vi "init.vi"(8 "error in (no error)":errorcluster, 11 "CL57RS in":refnum<class "CL57RS.lvclass">) -> (0 "error out":errorcluster, 3 "CL57RS out":refnum<class "CL57RS.lvclass">)   [LabVIEW 2025, in "Motor.lvlib" / "CL57RS.lvclass"]
uses:
  CL57RS.lvclass
  CL57RS.lvclass/CL57RS.ctl
  <vilib>/NI/Modbus Library/API/Wrapper/Create Serial Master.vi
  <vilib>/NI/Modbus Library/API/Wrapper/API Main.lvlib
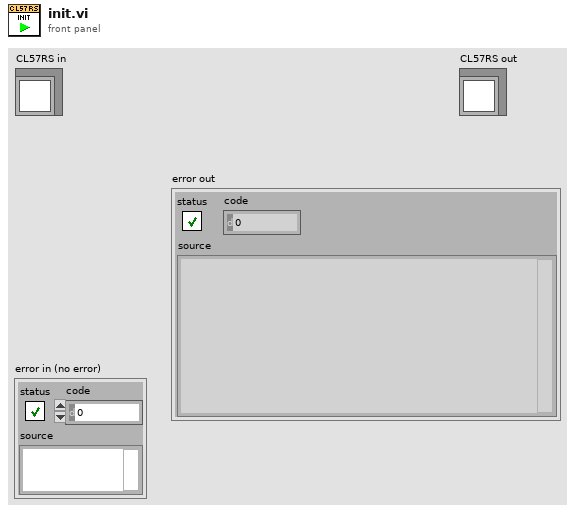
[diagram p1: front panel]
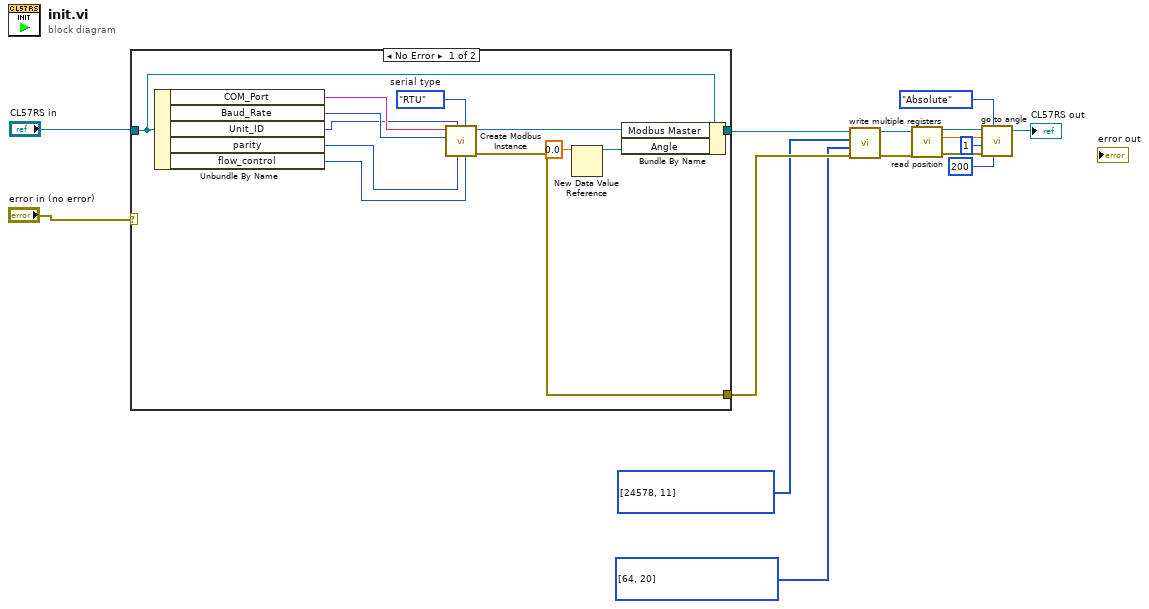
[diagram p0: block diagram]
diagram:
  n1 = case shown="No Error" "error in (no error)" {
    selector: "error in (no error)" -> [_ w29]
    tunnel: [w18 w29] -> w3
    tunnel: [w27 w28] -> w4
    tunnel: "CL57RS in" -> [w26 w28]
    frame No Error {
      w22 = enum16{"RTU", "ASCII"}."RTU"  # serial type
      n2 = Unbundle By Name(w26) -> ("COM_Port"=w25:string, "Baud_Rate"=w24:u32, "Unit_ID"=w23:u8, "parity"=w21:u16, "flow_control"=w20:u16)
      n3 = call-poly <vilib>:"Create Modbus Instance.vi"("flow control (none)"=w20, "serial type"=w22, "parity (even)"=w21, "unit ID"=w23, "baud rate"=w24, "VISA resource name"=w25) -> ("error out"=w18:errorcluster, "serial master instance"=w19:refnum<class "Modbus Master.lvclass">)  [unwired: 4 in]
      n4 = New Data Value Reference(data value=0.0) -> (data value reference=w17:refnum<data-value>)  [unwired: 1 in, 1 out]
      n5 = Bundle By Name(cluster=w26, "Modbus Master"=w19, "Angle"=w17) -> (w27:refnum<class "CL57RS.lvclass">)
    }
    frame Error {
    }
  }
  n6 = call "write multiple registers.vi"("error in (no error)"=w3, "register values"=u16[] [64, 20], "addresses"=u16[] [24578, 11], "CL57RS in"=w4) -> ("error out"=w5:errorcluster, "CL57RS out"=w6:refnum<class "CL57RS.lvclass">)  [unwired: 6 in]
  n7 = call-dynamic "read position.vi"("error in (no error)"=w5, "CL57RS in"=w6) -> ("error out"=w13:errorcluster, "Angle"=w12:dbl, "CL57RS out"=w10:refnum<class "CL57RS.lvclass">)  [unwired: 7 in]
  n8 = call-dynamic "go to angle.vi"("Pause Time [ms]"=200, "Relative?"=enum16{"Relative", "Absolute"}."Absolute", "error in (no error)"=w13, "Velocity [rpm]"=1, "Angle"=w12, "CL57RS in"=w10) -> ("CL57RS out"=→"CL57RS out":refnum<class "CL57RS.lvclass">)  [unwired: 4 in, 1 out]
